vi "表格指定单元格颜色变化.vi"() -> ()   [LabVIEW 2017]
uses:
  <vilib>/Utility/miscctls.llb/LVRowAndColumnTypeDef.ctl
panel:
  out "表格控件":string[][](table)
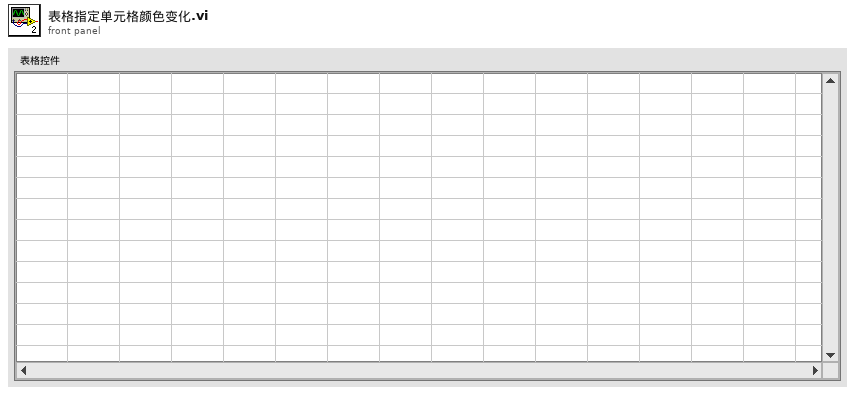
[diagram p1: front panel]
types:
  T1 = typedef "LVRowAndColumnTypeDef.ctl" = cluster{"Row":i32, "Column":i32}
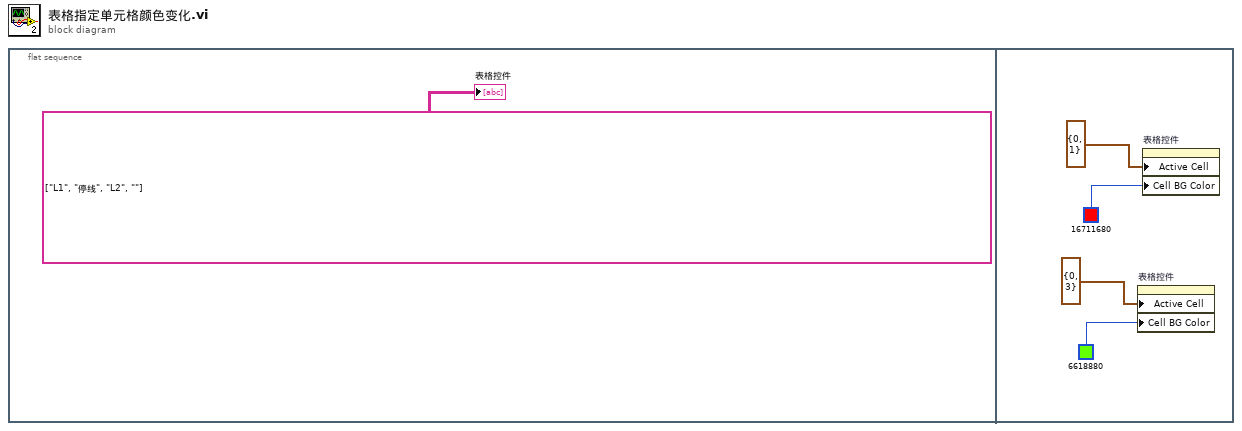
[diagram p0: block diagram]
diagram:
  n1 = flat-sequence {
    frame #0 {
      "表格控件" <- string[][] [["L1", "停线", "L2", ""]] ("项名")
    }
    frame #1 {
      n2 = property on="表格控件" class="Tbl (严格)"("Active Cell"=T1 {"Row"=0, "Column"=3} ("活动单元格:活动单元格"), "Cell BG Color"=u32 6618880) -> ()  [unwired: 2 in, 2 out]
      n3 = property on="表格控件" class="Tbl (严格)"("Active Cell"=T1 {"Row"=0, "Column"=1} ("活动单元格:活动单元格"), "Cell BG Color"=u32 16711680) -> ()  [unwired: 2 in, 2 out]
    }
  }
